vi "Entities for Target.vi"(10 "Target Name":string, 11 "Project Name":string) -> (3 "Entities":path[](array[path]))   [LabVIEW 2020, in "Conditum-Tools.lvlib" / "Entity Editor.lvclass"]
uses:
  Entity Editor.lvclass
  Conditum/Entity/Entity.lvclass
  NewEntityTemplate/NewEntityTemplate.lvclass
  Entity Editor.lvclass/Entity Editor.ctl
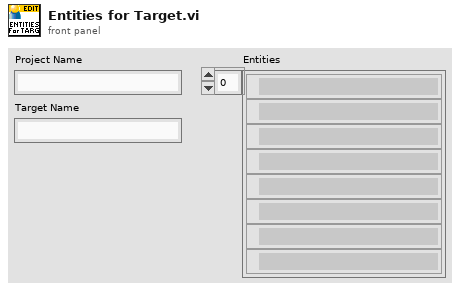
[diagram p1: front panel]
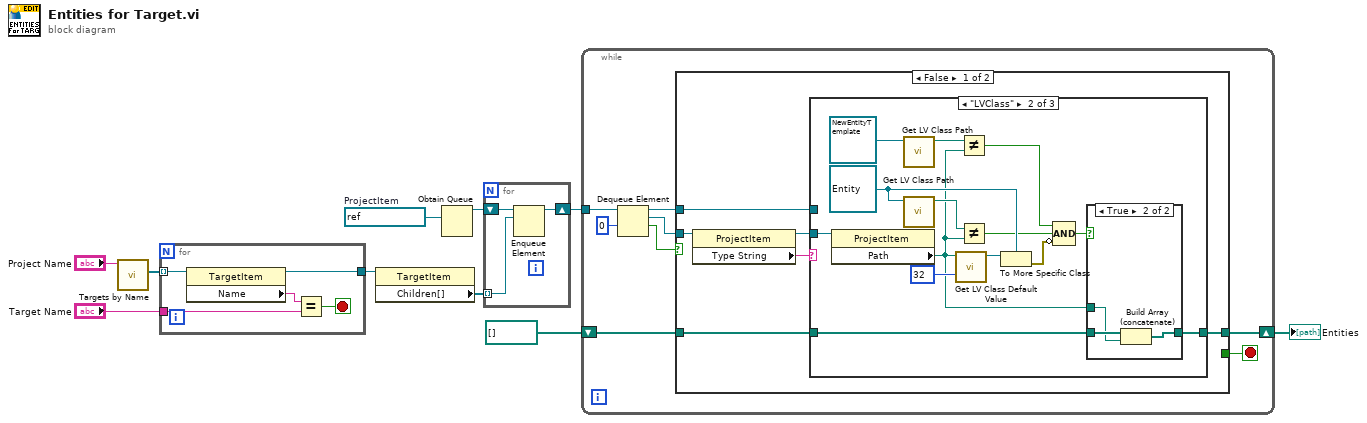
[diagram p0: block diagram]
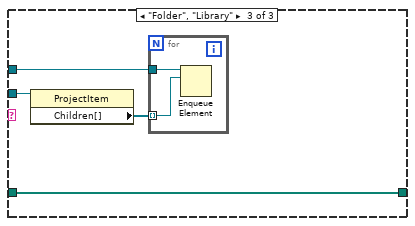
[diagram p4: hidden frame]
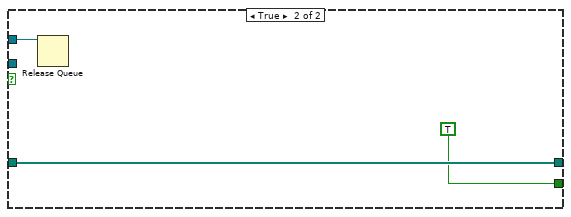
[diagram p5: hidden frame]
diagram:
  w6 = refnum<vi> refnum  # ProjectItem
  n1 = call "Targets by Name.vi"("Project Name"="Project Name") -> ("Targets"=w9:refnum<vi>[])  [unwired: 9 in, 1 out]
  n2 = for {
    tunnel: w9 -> [w15] mode=indexing
    tunnel: "Target Name" -> [w14]
    tunnel: [w12] -> w7
    stop <- w11 stop-if-true
    n3 = property class="TargetItem"(reference=w15) -> (reference out=w12:refnum<vi>, "Name"=w13:string)  [unwired: 1 in, 1 out]
    n4 = Equal?(x=w13, y=w14) -> (x = y?=w11:bool)
  }
  n5 = property class="TargetItem"(reference=w7) -> ("Children[]"=w5:refnum<vi>[])  [unwired: 1 in, 2 out]
  n6 = Obtain Queue(element data type=w6) -> (queue out=w4:refnum<queue>)  [unwired: 4 in, 2 out]
  n7 = for {
    tunnel: w5 -> [w17] mode=indexing
    shift-right: [w16] -> w3
    shift-left: w4 -> [w18]
    n8 = Enqueue Element(queue=w18, element=w17) -> (queue out=w16:refnum<queue>)  [unwired: 2 in, 2 out]
  }
  n9 = while {
    tunnel: w3 -> [w26]
    shift-right: [w20] -> w1
    shift-left: path[] [] -> [w21]
    stop <- w19 stop-if-true
    n10 = Dequeue Element(queue=w26, timeout in ms (-1)=0) -> (queue out=w22:refnum<queue>, element=w23:refnum<vi>, timed out?=w24:bool)  [unwired: 1 in, 1 out]
    n11 = case shown="False" w24 {
      tunnel: w23 -> [w32 _]
      tunnel: w22 -> [w31 w60]
      tunnel: w21 -> [w28 w59]
      tunnel: [w27 w59] -> w20
      tunnel: [_ TRUE] -> w19
      frame False {
        n12 = property class="ProjectItem"(reference=w32) -> (reference out=w29:refnum<vi>, "Type String"=w30:string)  [unwired: 1 in, 1 out]
        n13 = case shown="\"LVClass\"" w30 {
          tunnel: w31 -> [_ _ w53]
          tunnel: w29 -> [_ w47 w55]
          tunnel: w28 -> [w33 w44 w52]
          tunnel: [w33 w43 w52] -> w27
          frame Default {
          }
          frame "LVClass" {
            w42 = refnum<class "Entity.lvclass"> refnum ("Conditum:Entity")
            n14 = property class="ProjectItem"(reference=w47) -> ("Path"=w37:path)  [unwired: 1 in, 2 out]
            n15 = call <vilib>:"Get LV Class Path.vi"("object"=refnum<class "NewEntityTemplate.lvclass"> refnum ("Conditum-Tools.lvlib:NewEntityTemplate.lvclass")) -> ("class path"=w36:path)  [unwired: 9 in, 1 out]
            n16 = call <vilib>:"Get LV Class Path.vi"("object"=w42) -> ("class path"=w41:path)  [unwired: 9 in, 1 out]
            n17 = call <vilib>:"Get LV Class Default Value.vi"("options"=u32 32, "class path"=w37) -> ("object"=w45:refnum<class>)  [unwired: 8 in, 1 out]
            n18 = Not Equal?(x=w36, y=w37) -> (x != y?=w34:bool)
            n19 = Not Equal?(x=w41, y=w37) -> (x != y?=w35:bool)
            n20 = To More Specific Class(target class=w42, reference=w45) -> (error out=w40:errorcluster)  [unwired: 1 in, 1 out]
            n21 = Compound Arithmetic op=AND(w34, w35, invert w40) -> (w39:bool)
            n22 = case shown="True" w39 {
              tunnel: w37 -> [_ w50]
              tunnel: w44 -> [w48 w51]
              tunnel: [w48 w49] -> w43
              frame False {
              }
              frame True {
                n23 = Build Array (concatenate)(w51, w50) -> (w49:path[])
              }
            }
          }
          frame "Folder", "Library" {
            n24 = property class="ProjectItem"(reference=w55) -> ("Children[]"=w54:refnum<vi>[])  [unwired: 1 in, 2 out]
            n25 = for {
              tunnel: w54 -> [w56] mode=indexing
              tunnel: w53 -> [w57]
              n26 = Enqueue Element(queue=w57, element=w56) -> ()  [unwired: 2 in, 3 out]
            }
          }
        }
      }
      frame True {
        n27 = Release Queue(queue=w60) -> ()  [unwired: 2 in, 3 out]
      }
    }
  }
  "Entities" <- w1
